vi "Set Steer Commands (Absolute).vi"(8 "Rear Right":dbl, 9 "Rear Left":dbl, 10 "Front Right":dbl, 11 "Front Left":dbl) -> ()   [LabVIEW 2012]
uses:
  Globals/Jaguar Commands.vi
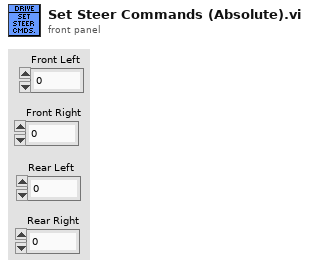
[diagram p1: front panel]
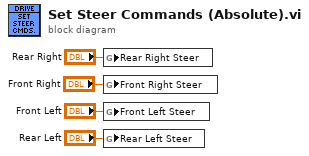
[diagram p0: block diagram]
diagram:
  n1 = global write "Jaguar Commands.vi" "Rear Right Steer"("Rear Right") -> ()
  n2 = global write "Jaguar Commands.vi" "Front Right Steer"("Front Right") -> ()
  n3 = global write "Jaguar Commands.vi" "Front Left Steer"("Front Left") -> ()
  n4 = global write "Jaguar Commands.vi" "Rear Left Steer"("Rear Left") -> ()
